vi "Elliptic Filter (CDB).vi"(0 "init/cont (init:F)":bool, 4 "order":i32=2, 5 "filter type":T1, 6 "stopband attenuation (dB)":dbl=60.0 format="%0.2f", 7 "passband ripple (dB)":dbl=1.0 format="%0.2f", 8 "low cutoff freq: fl":dbl=0.125 format="%0.4f", 9 "high cutoff freq: fh":dbl=0.45000000000000007 format="%0.2f", 10 "sampling freq: fs":dbl=1.0 format="%0.2f", 11 "X":cdb[](array[numeric])) -> (1 "error":i32, 3 "Filtered X":cdb[](array[numeric]))   [LabVIEW 2020, in "NI_AALBase.lvlib"]
doc: "Generates a digital elliptic filter by calling the Elliptic Coefficients VI. Wire data to the <B>X</B> input to determine the polymorphic instance to use or manually select the instance."
uses:
  <vilib>/Analysis/NI_AALBase.lvlib
  <vilib>/Analysis/3filter.llb/Filter Passband Type.ctl
  <vilib>/Analysis/baseanly.llb/IIR Cascade Filter (CDB).vi
panel:
  # "Elliptic Filter"
  # "Filter Controls"
  # "Frequency Controls"
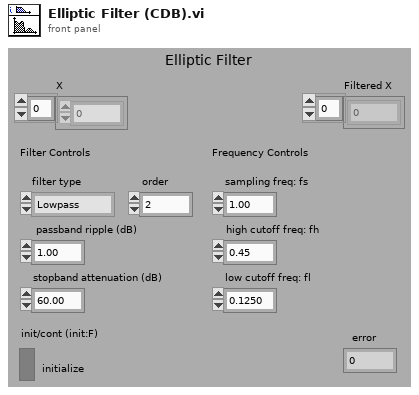
[diagram p1: front panel]
types:
  T1 = typedef "NI_AALBase.lvlib/Filter Passband Type.ctl" = enum32{"Lowpass", "Highpass", "Bandpass", "Bandstop"}
  T2 = cluster{"filter structure":enum32{"IIR 2nd Order", "IIR 4th Order"}, "Reverse Coefficients":dbl[], "Forward Coefficients":dbl[]}
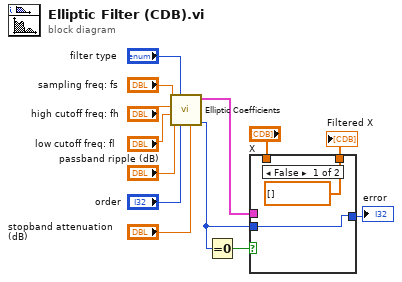
[diagram p0: block diagram]
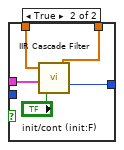
[diagram p2: hidden frame]
diagram:
  n1 = call <vilib>:"Elliptic Coefficients.vi"("stopband attenuation (dB)"="stopband attenuation (dB)", "order"="order", "filter type"="filter type", "passband ripple (dB)"="passband ripple (dB)", "low cutoff freq: fl"="low cutoff freq: fl", "high cutoff freq: fh"="high cutoff freq: fh", "sampling freq: fs"="sampling freq: fs") -> ("error"=w2:i32, "IIR Filter Cluster"=w3:T2)  [unwired: 3 in]
  n2 = Equal To 0?(x=w2) -> (x = 0?=w1:bool)
  n3 = case shown="False" w1 {
    tunnel: w2 -> [w15 _]
    tunnel: "X" -> [_ w16]
    tunnel: [cdb[] [] w19] -> w12
    tunnel: w3 -> [_ w17]
    tunnel: [w15 w20] -> w11
    frame False {
    }
    frame True {
      n4 = call-poly <vilib>:"IIR Cascade Filter.vi"("init/cont (init:F)"="init/cont (init:F)", "IIR Filter Cluster"=w17, "X"=w16) -> ("error"=w20:i32, "Filtered X"=w19:cdb[])
    }
  }
  "Filtered X" <- w12
  "error" <- w11
